vi "Get DC Voltage Offset.vi"(8 "error in (no error)":errorcluster, 11 "VISA resource name":refnum<visa-resource-name>) -> (0 "error out":errorcluster, 2 "Offset Value":dbl format="%^.3e", 3 "VISA resource name out":refnum<visa-resource-name>)   [LabVIEW 2011, in "Fluke 5XXX Series Multicalibrators.lvlib"]
doc: "This VI returns the value of dc offset applied to an ac output voltage.\n\nNote:\n\nThis VI is available only for instrument models 5500A and 5520A."
uses:
  Fluke 5XXX Series Multicalibrators.lvlib
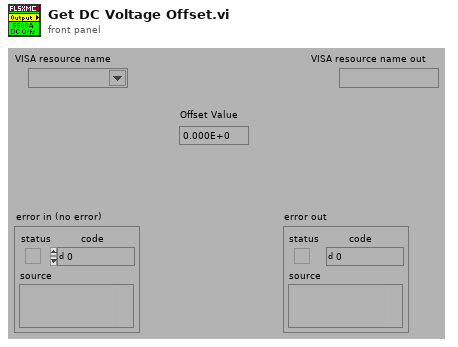
[diagram p1: front panel]
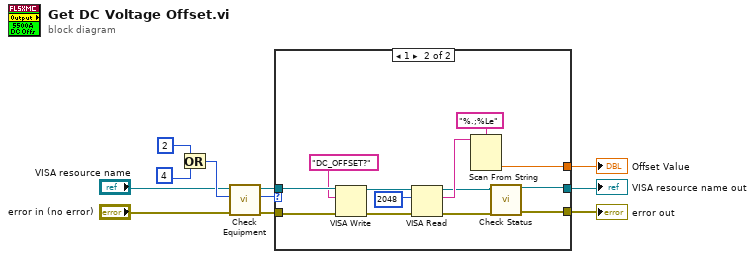
[diagram p0: block diagram]
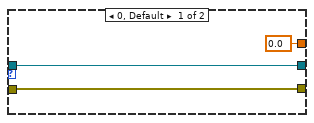
[diagram p2: hidden frame]
diagram:
  n1 = Or(x=2 ("Numeric"), y=4 ("Numeric")) -> (x .or. y?=w8:i32)
  n2 = call "Check Equipment.vi"("error in (no error)"="error in (no error)", "Bit Mask"=w8, "VISA resource name"="VISA resource name") -> ("error out"=w11:errorcluster, "Present?"=w10:u32, "VISA resource name out"=w9:refnum<visa-resource-name>)  [unwired: 6 in]
  n3 = case shown="1" w10 {
    tunnel: [w13 w26] -> w4
    tunnel: w11 -> [w14 w25]
    tunnel: w9 -> [w13 w24]
    tunnel: [w14 w27] -> w5
    tunnel: [0.0 w15] -> w1
    frame 0, Default {
    }
    frame 1 {
      n4 = VISA Write(VISA resource name=w24, write buffer="DC_OFFSET?", error in (no error)=w25) -> (VISA resource name out=w21:refnum<visa-resource-name>, error out=w20:errorcluster)  [unwired: 1 out]
      n5 = VISA Read(VISA resource name=w21, byte count=u32 2048 ("byte count (0)"), error in (no error)=w20) -> (VISA resource name out=w16:refnum<visa-resource-name>, read buffer=w17:string, error out=w18:errorcluster)  [unwired: 1 out]
      n6 = Scan From String(format string="%.;%Le", input string=w17) -> (output 1=w15:dbl)  [unwired: 3 in, 3 out]
      n7 = call "Check Status.vi"("VISA resource name"=w16, "error in (no error)"=w18) -> ("VISA resource name out"=w26:refnum<visa-resource-name>, "error out"=w27:errorcluster)  [unwired: 12 in]
    }
  }
  "Offset Value" <- w1
  "VISA resource name out" <- w4
  "error out" <- w5
